vi "Get Message Placement Cluster.vi"(6 "Is Serialization Cluster":bool=TRUE, 7 "MessageElementMetadata":T1, 8 "error in (no error)":errorcluster, 10 "typedef cluster":refnum<vi>, 11 "library in":refnum<vi>) -> (0 "error out":errorcluster, 1 "owning cluster":refnum<vi>, 2 "class data control":refnum<vi>, 3 "library out":refnum<vi>)   [LabVIEW 2019, in "gRPC Template Creation Utility.lvlib"]
uses:
  gRPC Template Creation Utility.lvlib
  TypeDefs/Message Element Metadata (Scripting).ctl
  TypeDefs/Message Element Type.ctl
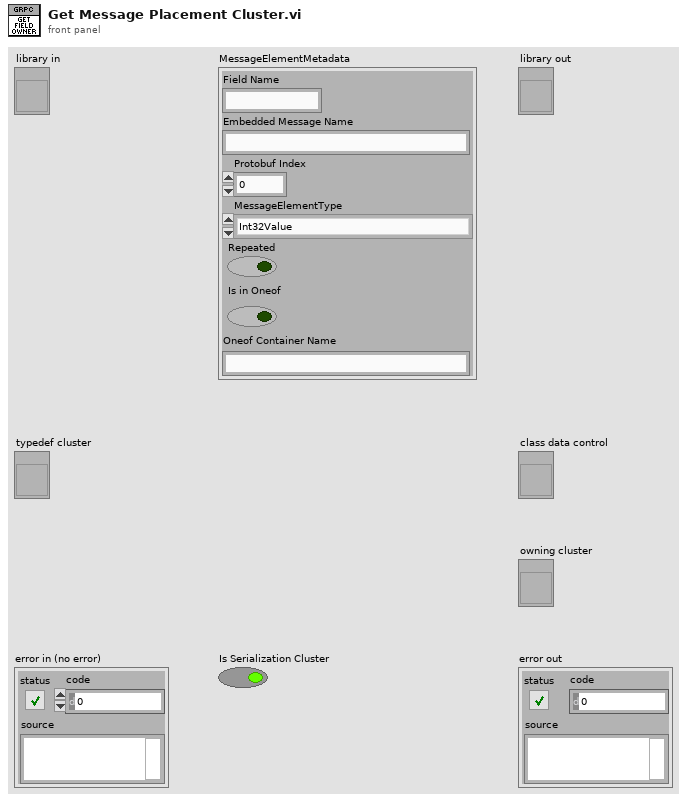
[diagram p1: front panel]
types:
  T1 = typedef "gRPC Template Creation Utility.lvlib/Message Element Metadata (Scripting).ctl" = cluster{"Field Name":string, "Embedded Message Name":string, "Protobuf Index":i32, "MessageElementType":T2, "Repeated":bool, "Is in Oneof":bool, "Oneof Container Name":string}
  T2 = typedef "gRPC Template Creation Utility.lvlib/Message Element Type.ctl" = enum32{"Int32Value", "FloatValue", "DoubleValue", "BoolValue", "StringValue", "MessageValue", "Int64Value", "UInt32Value", "UInt64Value", "EnumValue", "Bytes", "Fixed64", "Fixed32", "SFixed64", "SFixed32", "SInt64", "SInt32"}
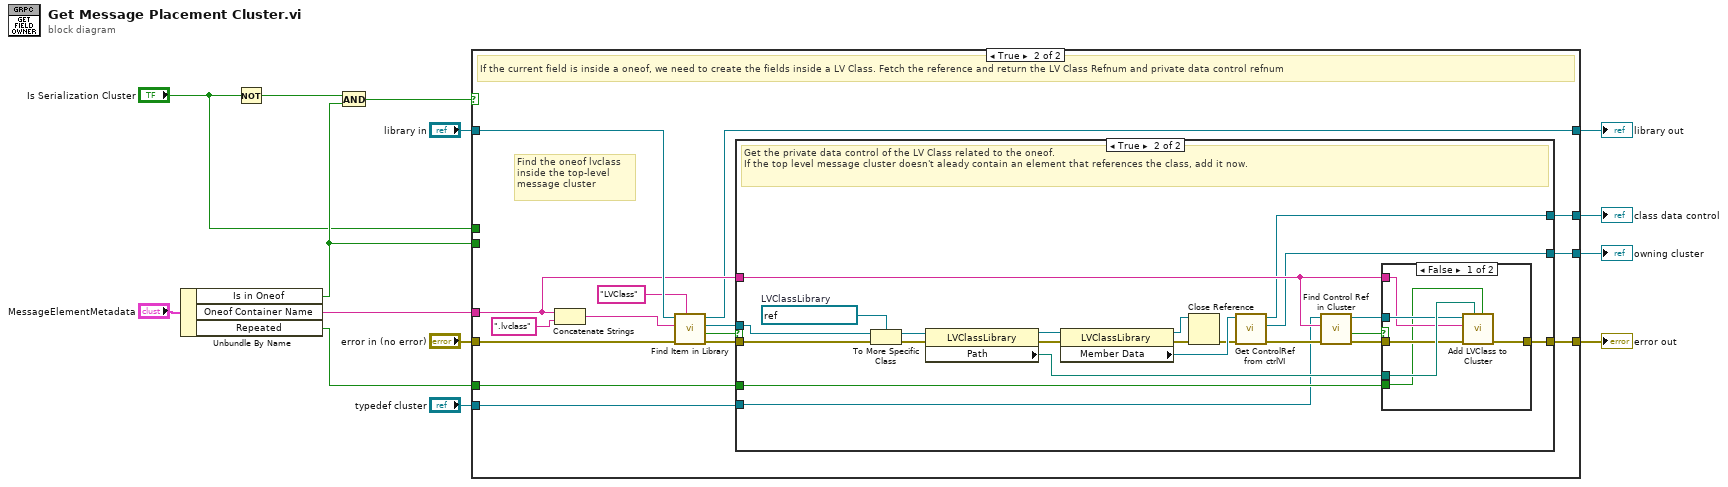
[diagram p0: block diagram]
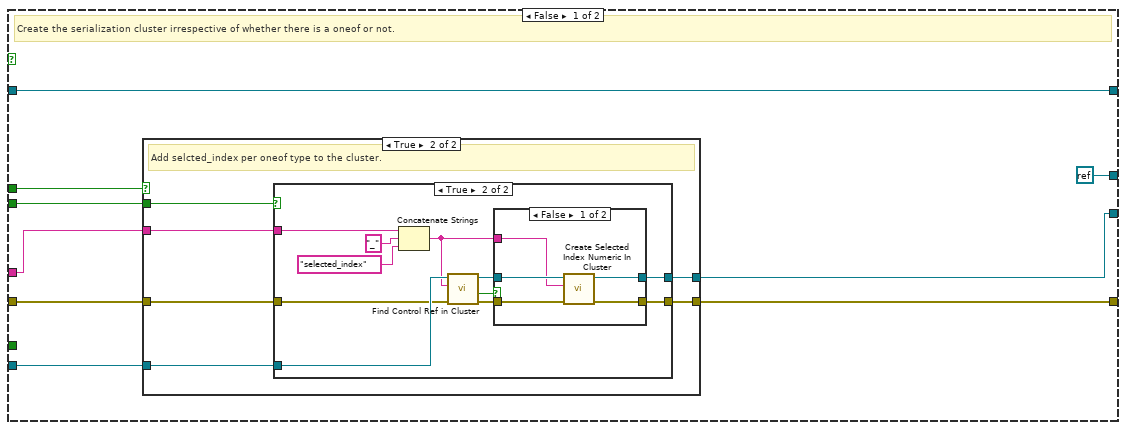
[diagram p2: hidden frame]
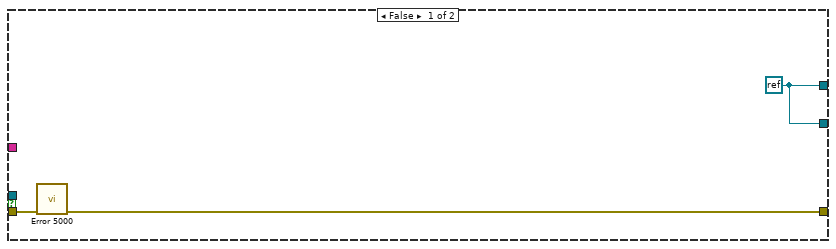
[diagram p6: hidden frame]
diagram:
  n1 = Unbundle By Name("MessageElementMetadata") -> ("Is in Oneof"=w5:bool, "Oneof Container Name"=w9:string, "Repeated"=w3:bool)
  n2 = Not(x="Is Serialization Cluster") -> (.not. x?=w6:bool)
  n3 = And(x=w6, y=w5) -> (x .and. y?=w7:bool)
  n4 = case shown="True" w7 {
    tunnel: w9 -> [w20 w59]
    tunnel: "error in (no error)" -> [w16 w65]
    tunnel: [w19 w57] -> w14
    tunnel: "library in" -> [w23 w66]
    tunnel: [w23 w56] -> w12
    tunnel: [w21 w55] -> w13
    tunnel: [refnum<k0> refnum w54] -> w2
    tunnel: w5 -> [w18 _]
    tunnel: "Is Serialization Cluster" -> [w17 _]
    tunnel: w3 -> [_ w53]
    tunnel: "typedef cluster" -> [w15 w52]
    frame False {
      # "Create the serialization cluster irrespective of whether there is a oneof or not."
      n5 = case shown="True" w17 {
        tunnel: [w24 w30] -> w21
        tunnel: w20 -> [_ w31]
        tunnel: w16 -> [w25 w27]
        tunnel: [w25 w29] -> w19
        tunnel: w18 -> [_ w28]
        tunnel: w15 -> [w24 w26]
        frame False {
        }
        frame True {
          # "Add selcted_index per oneof type to the cluster."
          n6 = case shown="True" w28 {
            tunnel: w26 -> [w32 w44]
            tunnel: w31 -> [_ w41]
            tunnel: [w32 w37] -> w30
            tunnel: w27 -> [w33 w35]
            tunnel: [w33 w34] -> w29
            frame False {
            }
            frame True {
              n7 = Concatenate Strings(w41, "_" ("string"), "selected_index" ("Control Name")) -> (w36:string)
              n8 = call "Find Control Ref in Cluster.vi"("error in (no error)"=w35, "Control Name"=w36, "Cluster ref in"=w44) -> ("error out"=w39:errorcluster, "Found ?"=w40:bool, "Cluster ref out"=w38:refnum<vi>)  [unwired: 5 in, 1 out]
              n9 = case shown="False" w40 {
                tunnel: w39 -> [w49 w51]
                tunnel: [w46 w51] -> w34
                tunnel: w38 -> [w48 w50]
                tunnel: [w47 w50] -> w37
                tunnel: w36 -> [w45 _]
                frame False {
                  n10 = call "Create Selected Index Numeric In Cluster.vi"("error in (no error)"=w49, "Label.Text"=w45, "Cluster in"=w48) -> ("error out"=w46:errorcluster, "Cluster out"=w47:refnum<vi>)  [unwired: 7 in]
                }
                frame True {
                }
              }
            }
          }
        }
      }
    }
    frame True {
      # "Find the oneof lvclass \ninside the top-level \nmessage cluster"
      # "If the current field is inside a oneof, we need to create the fields inside a LV Class. Fetch the reference and return the LV Class Refnum and private data control refnum"
      n11 = Concatenate Strings(w59, ".lvclass" ("string")) -> (w64:string)
      n12 = call "Find Item in Library.vi"("Item Type"="LVClass", "error in (no error)"=w65, "Item Name"=w64, "Library item in"=w66) -> ("error out"=w60:errorcluster, "Found?"=w62:bool, "Project Item (Library Item)"=w61:refnum<vi>, "Library item out"=w56:refnum<vi>)  [unwired: 4 in]
      n13 = case shown="True" w62 {
        tunnel: w61 -> [_ w89]
        tunnel: w60 -> [w68 w90]
        tunnel: w59 -> [_ w83]
        tunnel: [w67 w81] -> w57
        tunnel: [w69 w80] -> w55
        tunnel: [w69 w72] -> w54
        tunnel: w53 -> [_ w76]
        tunnel: w52 -> [_ w70]
        frame False {
          w69 = refnum<k0> refnum
          n14 = call "Error 5000.vi"("error in (no error)"=w68) -> ("error out"=w67:errorcluster)  [unwired: 10 in]
        }
        frame True {
          w88 = refnum<vi> refnum  # LVClassLibrary
          # "Get the private data control of the LV Class related to the oneof. \nIf the top level message cluster doesn't aleady contain an element that references the class, add it now."
          n15 = To More Specific Class(target class=w88, reference=w89, error in=w90) -> (specific class reference=w87:refnum<vi>, error out=w86:errorcluster)
          n16 = property class="LVClassLibrary"(reference=w87, error in=w86) -> (reference out=w85:refnum<vi>, error out=w84:errorcluster, "Path"=w91:path)
          n17 = property class="LVClassLibrary"(reference=w85, error in=w84) -> (reference out=w74:refnum<vi>, error out=w75:errorcluster, "Member Data"=w82:refnum<vi>)
          n18 = Close Reference(reference=w74, error in (no error)=w75) -> (error out=w73:errorcluster)
          n19 = call "Get ControlRef from ctrlVI.vi"("error in (no error)"=w73, "VI ref in"=w82) -> ("error out"=w71:errorcluster, "Control ref out"=w80:refnum<vi>, "VI ref out"=w72:refnum<vi>)  [unwired: 7 in]
          n20 = call "Find Control Ref in Cluster.vi"("error in (no error)"=w71, "Control Name"=w83, "Cluster ref in"=w70) -> ("error out"=w78:errorcluster, "Found ?"=w77:bool, "Cluster ref out"=w79:refnum<vi>)  [unwired: 5 in, 1 out]
          n21 = case shown="False" w77 {
            tunnel: w91 -> [w97 _]
            tunnel: [w96 w98] -> w81
            tunnel: w79 -> [w95 _]
            tunnel: w83 -> [w94 _]
            tunnel: w78 -> [w93 w98]
            tunnel: w76 -> [w92 _]
            frame False {
              n22 = call "Add LVClass to Cluster.vi"("isArray (F)"=w92, "LVClass path"=w97, "error in (no error)"=w93, "Field Name"=w94, "Owning cluster ref in"=w95) -> ("error out"=w96:errorcluster)  [unwired: 4 in, 2 out]
            }
            frame True {
            }
          }
        }
      }
    }
  }
  "error out" <- w14
  "owning cluster" <- w13
  "library out" <- w12
  "class data control" <- w2
